vi "InfluxWrite.vi"(8 "error in (no error)":errorcluster, 10 "input":dbl, 11 "name":string) -> (0 "error out":errorcluster)   [LabVIEW 2017]
uses:
  <vilib>/httpClient/POSTBuffer.vi
  <vilib>/httpClient/LabVIEWHTTPClient.lvlib
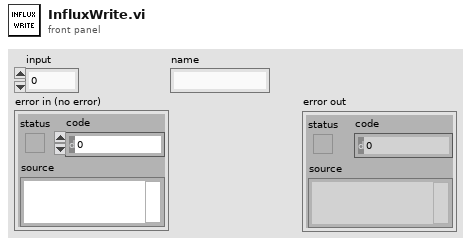
[diagram p1: front panel]
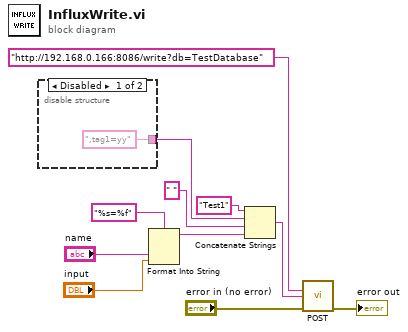
[diagram p0: block diagram]
diagram:
  n1 = disable-structure shown="Disabled" {
    disable-tunnel: [",tag1=yy" ("string") _] -> w9
    frame Disabled {
    }
    frame Enabled {
    }
  }
  n2 = Format Into String(format string="%s=%f", "name", "input") -> (resulting string=w6:string)  [unwired: 2 in, 1 out]
  n3 = Concatenate Strings("Test1" ("string"), w9, " " ("string"), w6) -> (w5:string)
  n4 = call-poly <vilib>:"POST.vi"("url"="http://192.168.0.166:8086/write?db=TestDatabase", "buffer"=w5, "error in (no error)"="error in (no error)") -> ("error out"=→"error out":errorcluster)  [unwired: 9 in, 3 out]
